vi "test_read-nmea-data2.vi"() -> ()   [LabVIEW 2019] (continued)
3,12,06,19,05,17,09,04,02,,,,,1.24,0.73,1.00,1*02\n\t\n15:12:20.33\tF9P\t$GNGSA,A,3,85,70,71,84,,,,,,,,,1.24,0.73,1.00,2*00\n\t\n15:12:20.35\tF9P\t$GNGSA,A,3,36,19,11,04,09,12,,,,,,,1.24,0.73,1.00,3*02\n\t\n15:12:20.37\tF9P\t$GNGSA,A,3,14,11,33,,,,,,,,,,1.24,0.73,1.00,4*03\n\t\n15:12:20.39\tF9P\t$GPGSV,3,1,09,02,55,319,20,04,18,043,29,05,37,247,28,06,64,049,37,1*62\n\t\n15:12:20.41\tF9P\t$GPGSV,3,2,09,09,45,074,30,12,23,276,31,17,33,154,36,19,52,157,35,1*6E\n\t\n15:12:20.43\tF9P\t$GPGSV,3,3,09,25,12,306,11,1*5C\n\t\n15:12:20.45\tF9P\t$GPGSV,3,1,09,02,55,319,,04,18,043,23,05,37,247,23,06,64,049,26,6*66\n\t\n15:12:20.47\tF9P\t$GPGSV,3,2,09,09,45,074,26,12,23,276,21,17,33,154,26,19,52,157,,6*68\n\t\n15:12:20.49\tF9P\t$GPGSV,3,3,09,25,12,306,,6*5B\n\t\n15:12:20.51\tF9P\t$GLGSV,2,1,08,69,12,031,,70,71,039,33,71,52,205,42,72,04,209,26,1*78\n\t\n15:12:20.53\tF9P\t$GLGSV,2,2,08,77,01,326,,84,20,122,08,85,70,067,40,86,37,330,,1*74\n\t\n15:12:20.55\tF9P\t$GLGSV,2,1,08,69,12,031,,70,71,039,,71,52,205,24,72,04,209,,3*7E\n\t\n15:12:20.57\tF9P\t$GLGSV,2,2,08,77,01,326,,84,20,122,13,85,70,067,23,86,37,330,,3*79\n\t\n15:12:20.59\tF9P\t$GAGSV,2,1,08,02,08,297,10,04,66,117,26,09,32,193,30,11,71,358,36,7*75\n\t\n15:12:20.61\tF9P\t$GAGSV,2,2,08,12,40,102,28,19,26,045,13,25,09,249,,36,26,308,15,7*75\n\t\n15:12:20.63\tF9P\t$GAGSV,2,1,08,02,08,297,,04,66,117,,09,32,193,,11,71,358,,2*73\n\t\n15:12:20.65\tF9P\t$GAGSV,2,2,08,12,40,102,,19,26,045,,25,09,249,,36,26,308,,2*7C\n\t\n15:12:20.67\tF9P\t$GBGSV,1,1,04,11,50,132,29,14,87,127,23,28,,,18,33,60,219,33,1*4C\n\t\n15:12:20.69\tF9P\t$GBGSV,1,1,03,11,50,132,30,14,87,127,,33,60,219,,3*43\n\t\n15:12:20.71\tF9P\t$GNGLL,3723.53875,N,12656.93680,E,061222.00,A,A*79\n\t\n15:12:20.73\tF9P\t\t\n15:12:20.75\tF9P\t\t\n15:12:20.77\tF9P\t\t\n15:12:20.79\tF9P\t\t\n15:12:20.81\tF9P\t\t\n15:12:20.83\tF9P\t\t\n15:12:20.85\tF9P\t\t\n15:12:20.87\tF9P\t\t\n15:12:20.89\tF9P\t\t\n15:12:20.91\tF9P\t\t\n15:12:20.93\tF9P\t\t\n15:12:20.95\tF9P\t\t\n15:12:20.97\tF9P\t\t\n15:12:20.99\tF9P\t\t\n15:12:21.01\tF9P\t\t\n15:12:21.03\tF9P\t\t\n15:12:21.05\tF9P\t\t\n15:12:21.07\tF9P\t\t\n15:12:21.09\tF9P\t\t\n15:12:21.11\tF9P\t\t\n15:12:21.13\tF9P\t\t\n15:12:21.15\tF9P\t\t\n15:12:21.17\tF9P\t\t\n15:12:21.19\tF9P\t\t\n15:12:21.21\tF9P\t\t\n15:12:21.23\tF9P\t\t\n15:12:21.25\tF9P\t$GNRMC,061223.00,A,3723.53919,N,12656.93709,E,1.332,46.74,250720,,,A,V*3E\n\t\n15:12:21.27\tF9P\t$GNVTG,46.74,T,,M,1.332,N,2.467,K,A*16\n\t\n15:12:21.29\tF9P\t$GNGGA,061223.00,3723.53919,N,12656.93709,E,1,12,0.86,40.3,M,18.5,M,,*70\n\t\n15:12:21.31\tF9P\t$GNGSA,A,3,12,06,19,05,17,09,04,02,,,,,1.43,0.86,1.14,1*0C\n\t\n15:12:21.33\tF9P\t$GNGSA,A,3,85,70,71,84,,,,,,,,,1.43,0.86,1.14,2*0E\n\t\n15:12:21.35\tF9P\t$GNGSA,A,3,36,19,11,04,09,12,,,,,,,1.43,0.86,1.14,3*0C\n\t\n15:12:21.37\tF9P\t$GNGSA,A,3,14,11,33,,,,,,,,,,1.43,0.86,1.14,4*0D\n\t\n15:12:21.39\tF9P\t$GPGSV,3,1,09,02,55,319,20,04,18,043,27,05,37,247,36,06,64,049,36,1*62\n\t\n15:12:21.41\tF9P\t$GPGSV,3,2,09,09,45,074,30,12,23,276,30,17,33,154,33,19,52,157,30,1*6F\n\t\n15:12:21.43\tF9P\t$GPGSV,3,3,09,25,12,306,,1*5C\n\t\n15:12:21.45\tF9P\t$GPGSV,3,1,09,02,55,319,,04,18,043,22,05,37,247,24,06,64,049,27,6*61\n\t\n15:12:21.47\tF9P\t$GPGSV,3,2,09,09,45,074,25,12,23,276,20,17,33,154,25,19,52,157,,6*69\n\t\n15:12:21.49\tF9P\t$GPGSV,3,3,09,25,12,306,,6*5B\n\t\n15:12:21.51\tF9P\t$GLGSV,2,1,08,69,12,031,,70,71,039,30,71,52,205,39,72,04,209,25,1*74\n\t\n15:12:21.53\tF9P\t$GLGSV,2,2,08,77,01,326,,84,20,122,12,85,70,067,33,86,37,330,,1*7B\n\t\n15:12:21.55\tF9P\t$GLGSV,2,1,08,69,12,031,,70,71,039,,71,52,205,25,72,04,209,,3*7F\n\t\n15:12:21.57\tF9P\t$GLGSV,2,2,08,77,01,326,,84,20,122,12,85,70,067,21,86,37,330,,3*7A\n\t\n15:12:21.59\tF9P\t$GAGSV,2,1,08,02,08,297,08,04,66,117,34,09,32,193,30,11,71,358,37,7*7E\n\t\n15:12:21.61\tF9P\t$GAGSV,2,2,08,12,40,102,29,19,26,045,12,25,09,249,,36,26,308,14,7*74\n\t\n15:12:21.63\tF9P\t$GAGSV,2,1,08,02,08,297,,04,66,117,,09,32,193,,11,71,358,32,2*72\n\t\n15:12:21.65\tF9P\t$GAGSV,2,2,08,12,40,102,,19,26,045,,25,09,249,,36,26,308,,2*7C\n\t\n15:12:21.67\tF9P\t$GBGSV,1,1,04,11,50,132,28,14,87,127,24,28,,,17,33,60,219,33,1*45\n\t\n15:12:21.69\tF9P\t$GBGSV,1,1,03,11,50,132,,14,87,127,,33,60,219,,3*40\n\t\n15:12:21.71\tF9P\t$GNGLL,3723.53919,N,12656.93709,E,061223.00,A,A*73\n\t\n15:12:21.73\tF9P\t\t\n15:12:21.75\tF9P\t\t\n15:12:21.77\tF9P\t\t\n15:12:21.79\tF9P\t\t\n15:12:21.81\tF9P\t\t\n15:12:21.83\tF9P\t\t\n15:12:21.85\tF9P\t\t\n15:12:21.87\tF9P\t\t\n15:12:21.89\tF9P\t\t\n15:12:21.91\tF9P\t\t\n15:12:21.93\tF9P\t\t\n15:12:21.95\tF9P\t\t\n15:12:21.97\tF9P\t\t\n15:12:21.99\tF9P\t\t\n15:12:22.01\tF9P\t\t\n15:12:22.03\tF9P\t\t\n15:12:22.05\tF9P\t\t\n15:12:22.07\tF9P\t\t\n15:12:22.09\tF9P\t\t\n15:12:22.11\tF9P\t\t\n15:12:22.13\tF9P\t\t\n15:12:22.15\tF9P\t\t\n15:12:22.17\tF9P\t\t\n15:12:22.19\tF9P\t\t\n15:12:22.21\tF9P\t\t\n15:12:22.23\tF9P\t$GNRMC,061224.00,A,3723.53944,N,12656.93745,E,1.337,51.42,250720\t\n15:12:22.25\tF9P\t,,,A,V*3F\n\t\n15:12:22.27\tF9P\t$GNVTG,51.42,T,,M,1.337,N,2.476,K,A*10\n\t\n15:12:22.29\tF9P\t$GNGGA,061224.00,3723.53944,N,12656.93745,E,1,12,0.73,40.9,M,18.5,M,,*77\n\t\n15:12:22.31\tF9P\t$GNGSA,A,3,12,06,19,05,17,09,04,02,,,,,1.26,0.73,1.03,1*03\n\t\n15:12:22.33\tF9P\t$GNGSA,A,3,85,70,71,84,,,,,,,,,1.26,0.73,1.03,2*01\n\t\n15:12:22.35\tF9P\t$GNGSA,A,3,36,19,11,04,09,12,,,,,,,1.26,0.73,1.03,3*03\n\t\n15:12:22.37\tF9P\t$GNGSA,A,3,14,11,33,,,,,,,,,,1.26,0.73,1.03,4*02\n\t\n15:12:22.39\tF9P\t$GPGSV,3,1,09,02,55,319,20,04,18,043,31,05,37,247,31,06,64,049,28,1*6D\n\t\n15:12:22.41\tF9P\t$GPGSV,3,2,09,09,45,074,28,12,23,276,30,17,33,154,30,19,52,157,36,1*63\n\t\n15:12:22.43\tF9P\t$GPGSV,3,3,09,25,12,306,,1*5C\n\t\n15:12:22.45\tF9P\t$GPGSV,3,1,09,02,55,319,,04,18,043,20,05,37,247,24,06,64,049,26,6*62\n\t\n15:12:22.47\tF9P\t$GPGSV,3,2,09,09,45,074,25,12,23,276,19,17,33,154,26,19,52,157,,6*60\n\t\n15:12:22.49\tF9P\t$GPGSV,3,3,09,25,12,306,,6*5B\n\t\n15:12:22.51\tF9P\t$GLGSV,2,1,08,69,12,031,,70,71,039,33,71,52,205,30,72,04,209,23,1*78\n\t\n15:12:22.53\tF9P\t$GLGSV,2,2,08,77,01,326,,84,20,122,10,85,70,067,35,86,37,330,,1*7F\n\t\n15:12:22.55\tF9P\t$GLGSV,2,1,08,69,12,031,,70,71,039,,71,52,205,24,72,04,209,,3*7E\n\t\n15:12:22.57\tF9P\t$GLGSV,2,2,08,77,01,326,,84,20,122,11,85,70,067,21,86,37,330,,3*79\n\t\n15:12:22.59\tF9P\t$GAGSV,2,1,08,02,08,297,07,04,66,117,31,09,32,193,31,11,71,358,37,7*75\n\t\n15:12:22.61\tF9P\t$GAGSV,2,2,08,12,40,102,29,19,26,045,11,25,09,249,,36,26,308,14,7*77\n\t\n15:12:22.63\tF9P\t$GAGSV,2,1,08,02,08,297,,04,66,117,29,09,32,193,,11,71,358,,2*78\n\t\n15:12:22.65\tF9P\t$GAGSV,2,2,08,12,40,102,,19,26,045,,25,09,249,,36,26,308,,2*7C\n\t\n15:12:22.67\tF9P\t$GBGSV,1,1,04,11,50,132,29,14,87,127,30,28,,,18,33,60,219,29,1*45\n\t\n15:12:22.69\tF9P\t$GBGSV,1,1,03,11,50,132,29,14,87,127,,33,60,219,,3*4B\n\t\n15:12:22.71\tF9P\t$GNGLL,3723.53944,N,12656.93745,E,061224.00,A,A*74\n\t\n15:12:22.73\tF9P\t\t\n15:12:22.75\tF9P\t\t\n15:12:22.77\tF9P\t\t\n15:12:22.79\tF9P\t\t\n15:12:22.81\tF9P\t\t\n15:12:22.83\tF9P\t\t\n15:12:22.85\tF9P\t\t\n15:12:22.87\tF9P\t\t\n15:12:22.89\tF9P\t\t\n15:12:22.91\tF9P\t\t\n15:12:22.93\tF9P\t\t\n15:12:22.95\tF9P\t\t\n15:12:22.97\tF9P\t\t\n15:12:22.99\tF9P\t\t\n15:12:23.01\tF9P\t\t\n15:12:23.03\tF9P\t\t\n15:12:23.05\tF9P\t\t\n15:12:23.07\tF9P\t\t\n15:12:23.09\tF9P\t\t\n15:12:23.11\tF9P\t\t\n15:12:23.13\tF9P\t\t\n15:12:23.15\tF9P\t\t\n15:12:23.17\tF9P\t\t\n15:12:23.19\tF9P\t\t\n15:12:23.21\tF9P\t\t\n15:12:23.23\tF9P\t$GNRMC,061225.00,A,3723.53964,N,12656.93801,E,1.830,59.59,250720,,,A,V*3D\n\t\n15:12:23.25\tF9P\t$GNVTG,59.59,T,,M,1.830,N,3.389,K,A*18\n\t\n15:12:23.27\tF9P\t$GNGGA,061225.00,3723.53964,N,12656.93801,E,1,12,0.74,41.4,M,18.5,M,,*70\n\t\n15:12:23.29\tF9P\t$GNGSA,A,3,12,06,19,05,17,09,04,02,,,,,1.27,0.74,1.04,1*02\n\t\n15:12:23.31\tF9P\t$GNGSA,A,3,85,70,71,84,,,,,,,,,1.27,0.74,1.04,2*00\n\t\n15:12:23.33\tF9P\t$GNGSA,A,3,36,19,11,04,09,12,,,,,,,1.27,0.74,1.04,3*02\n\t\n15:12:23.35\tF9P\t$GNGSA,A,3,14,11,33,,,,,,,,,,1.27,0.74,1.04,4*03\n\t\n15:12:23.37\tF9P\t$GPGSV,3,1,09,02,55,319,21,04,18,043,24,05,37,247,27,06,64,049,29,1*6E\n\t\n15:12:23.39\tF9P\t$GPGSV,3,2,09,09,45,074,34,12,23,276,29,17,33,154,32,19,52,157,32,1*60\n\t\n15:12:23.41\tF9P\t$GPGSV,3,3,09,25,12,306,,1*5C\n\t\n15:12:23.43\tF9P\t$GPGSV,3,1,09,02,55,319,,04,18,043,21,05,37,247,24,06,64,049,26,6*63\n\t\n15:12:23.45\tF9P\t$GPGSV,3,2,09,09,45,074,26,12,23,276,19,17,33,154,25,19,52,157,,6*60\n\t\n15:12:23.47\tF9P\t$GPGSV,3,3,09,25,12,306,,6*5B\n\t\n15:12:23.49\tF9P\t$GLGSV,2,1,08,69,12,031,,70,71,039,29,71,52,205,40,72,04,209,24,1*73\n\t\n15:12:23.51\tF9P\t$GLGSV,2,2,08,77,01,326,,84,20,122,08,85,70,067,34,86,37,330,,1*77\n\t\n15:12:23.53\tF9P\t$GLGSV,2,1,08,69,12,031,,70,71,039,,71,52,205,23,72,04,209,,3*79\n\t\n15:12:23.55\tF9P\t$GLGSV,2,2,08,77,01,326,,84,20,122,11,85,70,067,23,86,37,330,,3*7B\n\t\n15:12:23.57\tF9P\t$GAGSV,2,1,08,02,08,297,12,04,66,117,31,09,32,193,35,11,71,358,32,7*70\n\t\n15:12:23.59\tF9P\t$GAGSV,2,2,08,12,40,102,29,19,26,045,11,25,09,249,,36,26,308,15,7*76\n\t\n15:12:23.61\tF9P\t$GAGSV,2,1,08,02,08,297,,04,66,117,,09,32,193,,11,71,358,33,2*73\n\t\n15:12:23.63\tF9P\t$GAGSV,2,2,08,12,40,102,,19,26,045,,25,09,249,,36,26,308,,2*7C\n\t\n15:12:23.65\tF9P\t$GBGSV,1,1,04,11,50,132,29,14,87,127,30,28,,,18,33,60,219,33,1*4E\n\t\n15:12:23.67\tF9P\t$GBGSV,1,1,03,11,50,132,,14,87,127,,33,60,219,,3*40\n\t\n15:12:23.69\tF9P\t$GNGLL,3723.53964,N,12656.93801,E,061225.00,A,A*78\n\t\n15:12:23.71\tF9P\t\t\n15:12:23.73\tF9P\t\t\n15:12:23.75\tF9P\t\t\n15:12:23.77\tF9P\t\t\n15:12:23.79\tF9P\t\t\n15:12:23.81\tF9P\t\t\n15:12:23.83\tF9P\t\t\n15:12:23.85\tF9P\t\t\n15:12:23.87\tF9P\t\t\n15:12:23.89\tF9P\t\t\n15:12:23.91\tF9P\t\t\n15:12:23.93\tF9P\t\t\n15:12:23.95\tF9P\t\t\n15:12:23.97\tF9P\t\t\n15:12:23.99\tF9P\t\t\n15:12:24.01\tF9P\t\t\n15:12:24.03\tF9P\t\t\n15:12:24.05\tF9P\t\t\n15:12:24.07\tF9P\t\t\n15:12:24.09\tF9P\t\t\n15:12:24.11\tF9P\t\t\n15:12:24.13\tF9P\t\t\n15:12:24.15\tF9P\t\t\n15:12:24.17\tF9P\t\t\n15:12:24.19\tF9P\t\t\n15:12:24.21\tF9P\t\t\n15:12:24.23\tF9P\t$GNRMC,061226.00,A,3723.53985,N,12656.93886,E,2.379,68.89,250720,,,A,V*34\n\t\n15:12:24.25\tF9P\t$GNVTG,68.89,T,,M,2.379,N,4.406,K,A*15\n\t\n15:12:24.27\tF9P\t$GNGGA,061226.00,3723.53985,N,12656.93886,E,1,12,0.73,41.5,M,18.5,M,,*75\n\t\n15:12:24.29\tF9P\t$GNGSA,A,3,12,06,19,05,17,09,04,02,,,,,1.24,0.73,1.00,1*02\n\t\n15:12:24.31\tF9P\t$GNGSA,A,3,85,70,71,84,,,,,,,,,1.24,0.73,1.00,2*00\n\t\n15:12:24.33\tF9P\t$GNGSA,A,3,36,19,11,04,09,12,,,,,,,1.24,0.73,1.00,3*02\n\t\n15:12:24.35\tF9P\t$GNGSA,A,3,14,11,33,,,,,,,,,,1.24,0.73,1.00,4*03\n\t\n15:12:24.37\tF9P\t$GPGSV,3,1,09,02,55,319,20,04,18,043,26,05,37,247,33,06,64,049,29,1*68\n\t\n15:12:24.39\tF9P\t$GPGSV,3,2,09,09,45,074,29,12,23,276,28,17,33,154,35,19,52,157,32,1*6A\n\t\n15:12:24.41\tF9P\t$GPGSV,3,3,09,25,12,306,,1*5C\n\t\n15:12:24.43\tF9P\t$GPGSV,3,1,09,02,55,319,,04,18,043,22,05,37,247,24,06,64,049,27,6*61\n\t\n15:12:24.45\tF9P\t$GPGSV,3,2,09,09,45,074,31,12,23,276,19,17,33,154,27,19,52,157,,6*64\n\t\n15:12:24.47\tF9P\t$GPGSV,3,3,09,25,12,306,,6*5B\n\t\n15:12:24.49\tF9P\t$GLGSV,2,1,08,69,12,031,,70,71,039,29,71,52,205,43,72,04,209,25,1*71\n\t\n15:12:24.51\tF9P\t$GLGSV,2,2,08,77,01,326,,84,20,122,12,85,70,067,35,86,37,330,,1*7D\n\t\n15:12:24.53\tF9P\t$GLGSV,2,1,08,69,12,031,,70,71,039,,71,52,205,30,72,04,209,,3*7B\n\t\n15:12:24.55\tF9P\t$GLGSV,2,2,08,77,01,326,,84,20,122,11,85,70,067,22,86,37,330,,3*7A\n\t\n15:12:24.57\tF9P\t$GAGSV,2,1,08,02,08,297,10,04,66,117,30,09,32,193,38,11,71,358,32,7*7E\n\t\n15:12:24.59\tF9P\t$GAGSV,2,2,08,12,40,102,29,19,26,045,13,25,09,249,,36,26,308,15,7*74\n\t\n15:12:24.61\tF9P\t$GAGSV,2,1,08,02,08,297,,04,66,117,,09,32,193,,11,71,358,,2*73\n\t\n15:12:24.63\tF9P\t$GAGSV,2,2,08,12,40,102,,19,26,045,,25,09,249,,36,26,308,,2*7C\n\t\n15:12:24.65\tF9P\t$GBGSV,1,1,04,11,50,132,30,14,87,127,30,28,,,18,33,60,219,28,1*4C\n\t\n15:12:24.67\tF9P\t$GBGSV,1,1,03,11,50,132,,14,87,127,,33,60,219,,3*40\n\t\n15:12:24.69\tF9P\t$GNGLL,3723.53985,N,12656.93886,E,061226.00,A,A*7B\n\t\n15:12:24.71\tF9P\t\t\n15:12:24.73\tF9P\t\t\n15:12:24.75\tF9P\t\t\n15:12:24.77\tF9P\t\t\n15:12:24.79\tF9P\t\t\n15:12:24.81\tF9P\t\t\n15:12:24.83\tF9P\t\t\n15:12:24.85\tF9P\t\t\n15:12:24.87\tF9P\t\t\n15:12:24.89\tF9P\t\t\n15:12:24.91\tF9P\t\t\n15:12:24.93\tF9P\t\t\n15:12:24.95\tF9P\t\t\n15:12:24.97\tF9P\t\t\n15:12:24.99\tF9P\t\t\n15:12:25.01\tF9P\t\t\n15:12:25.03\tF9P\t\t\n15:12:25.05\tF9P\t\t\n15:12:25.07\tF9P\t\t\n15:12:25.09\tF9P\t\t\n15:12:25.11\tF9P\t\t\n15:12:25.13\tF9P\t\t\n15:12:25.15\tF9P\t\t\n15:12:25.17\tF9P\t\t\n15:12:25.19\tF9P\t\t\n15:12:25.21\tF9P\t\t\n15:12:25.23\tF9P\t$GNRMC,061227.00,A,3723.53985,N,12656.93969,E,2.036,75.18,250720,,,A,V*39\n\t\n15:12:25.25\tF9P\t$GNVTG,75.18,T,,M,2.036,N,3.770,K,A*1C\n\t\n15:12:25.27\tF9P\t$GNGGA,061227.00,3723.53985,N,12656.93969,E,1,12,0.93,41.9,M,18.5,M,,*76\n\t\n15:12:25.29\tF9P\t$GNGSA,A,3,12,06,19,05,17,09,04,02,,,,,1.55,0.93,1.24,1*0C\n\t\n15:12:25.31\tF9P\t$GNGSA,A,3,85,70,71,84,,,,,,,,,1.55,0.93,1.24,2*0E\n\t\n15:12:25.33\tF9P\t$GNGSA,A,3,36,19,11,04,09,12,,,,,,,1.55,0.93,1.24,3*0C\n\t\n15:12:25.35\tF9P\t$GNGSA,A,3,14,11,33,,,,,,,,,,1.55,0.93,1.24,4*0D\n\t\n15:12:25.37\tF9P\t$GPGSV,3,1,09,02,55,319,20,04,18,043,26,05,37,247,36,06,64,049,33,1*66\n\t\n15:12:25.39\tF9P\t$GPGSV,3,2,09,09,45,074,28,12,23,276,28,17,33,154,34,19,52,157,32,1*6A\n\t\n15:12:25.41\tF9P\t$GPGSV,3,3,09,25,12,306,,1*5C\n\t\n15:12:25.43\tF9P\t$GPGSV,3,1,09,02,55,319,,04,18,043,21,05,37,247,25,06,64,049,26,6*62\n\t\n15:12:25.45\tF9P\t$GPGSV,3,2,09,09,45,074,23,12,23,276,21,17,33,154,27,19,52,157,,6*6C\n\t\n15:12:25.47\tF9P\t$GPGSV,3,3,09,25,12,306,,6*5B\n\t\n15:12:25.49\tF9P\t$GLGSV,2,1,08,69,12,031,,70,71,039,29,71,52,205,42,72,04,209,26,1*73\n\t\n15:12:25.51\tF9P\t$GLGSV,2,2,08,77,01,326,,84,20,122,10,85,70,067,32,86,37,330,,1*78\n\t\n15:12:25.53\tF9P\t$GLGSV,2,1,08,69,12,031,,70,71,039,,71,52,205,30,72,04,209,,3*7B\n\t\n15:12:25.55\tF9P\t$GLGSV,2,2,08,77,01,326,,84,20,122,09,85,70,067,23,86,37,330,,3*72\n\t\n15:12:25.57\tF9P\t$GAGSV,2,1,08,02,08,297,10,04,66,116,29,09,32,193,38,11,71,358,27,7*73\n\t\n15:12:25.59\tF9P\t$GAGSV,2,2,08,12,40,102,30,19,26,045,15,25,09,249,,36,26,308,14,7*7B\n\t\n15:12:25.61\tF9P\t$GAGSV,2,1,08,02,08,297,,04,66,116,,09,32,193,,11,71,358,,2*72\n\t\n15:12:25.63\tF9P\t$GAGSV,2,2,08,12,40,102,,19,26,045,,25,09,249,,36,26,308,,2*7C\n\t\n15:12:25.65\tF9P\t$GBGSV,1,1,04,11,50,132,28,14,87,127,30,28,,,18,33,60,219,28,1*45\n\t\n15:12:25.67\tF9P\t$GBGSV,1,1,03,11,50,132,,14,87,127,,33,60,219,,3*40\n\t\n15:12:25.69\tF9P\t$GNGLL,3723.53985,N,12656.93969,E,061227.00,A,A*7A\n\t\n15:12:25.71\tF9P\t\t\n15:12:25.73\tF9P\t\t\n15:12:25.75\tF9P\t\t\n15:12:25.77\tF9P\t\t\n15:12:25.79\tF9P\t\t\n15:12:25.81\tF9P\t\t\n15:12:25.83\tF9P\t\t\n15:12:25.85\tF9P\t\t\n15:12:25.87\tF9P\t\t\n15:12:25.89\tF9P\t\t\n15:12:25.91\tF9P\t\t\n15:12:25.93\tF9P\t\t\n15:12:25.95\tF9P\t\t\n15:12:25.97\tF9P\t\t\n15:12:25.99\tF9P\t\t\n15:12:26.01\tF9P\t\t\n15:12:26.03\tF9P\t\t\n15:12:26.05\tF9P\t\t\n15:12:26.07\tF9P\t\t\n15:12:26.09\tF9P\t\t\n15:12:26.11\tF9P\t\t\n15:12:26.13\tF9P\t\t\n15:12:26.15\tF9P\t\t\n15:12:26.17\tF9P\t\t\n15:12:26.19\tF9P\t\t\n15:12:26.21\tF9P\t\t\n15:12:26.23\tF9P\t$GNRMC,061228.00,A,3723.54009,N,12656.94073,E,2.854,71.20,250720,,,A,V*3A\n\t\n15:12:26.25\tF9P\t$GNVTG,71.20,T,,M,2.854,N,5.286,K,A*15\n\t\n15:12:26.27\tF9P\t$GNGGA,061228.00,3723.54009,N,12656.94073,E,1,12,0.75,41.7,M,18.5,M,,*70\n\t\n15:12:26.29\tF9P\t$GNGSA,A,3,12,06,19,05,17,09,04,02,,,,,1.29,0.75,1.04,1*0D\n\t\n15:12:26.31\tF9P\t$GNGSA,A,3,85,70,71,84,,,,,,,,,1.29,0.75,1.04,2*0F\n\t\n15:12:26.33\tF9P\t$GNGSA,A,3,36,19,11,04,09,12,,,,,,,1.29,0.75,1.04,3*0D\n\t\n15:12:26.35\tF9P\t$GNGSA,A,3,14,11,33,,,,,,,,,,1.29,0.75,1.04,4*0C\n\t\n15:12:26.37\tF9P\t$GPGSV,3,1,09,02,55,319,20,04,18,043,25,05,37,247,44,06,64,049,30,1*63\n\t\n15:12:26.39\tF9P\t$GPGSV,3,2,09,09,45,074,27,12,23,276,27,17,33,154,34,19,52,157,26,1*6F\n\t\n15:12:26.41\tF9P\t$GPGSV,3,3,09,25,12,306,,1*5C\n\t\n15:12:26.43\tF9P\t$GPGSV,3,1,09,02,55,319,,04,18,043,21,05,37,247,25,06,64,049,26,6*62\n\t\n15:12:26.45\tF9P\t$GPGSV,3,2,09,09,45,074,25,12,23,276,21,17,33,154,27,19,52,157,,6*6A\n\t\n15:12:26.47\tF9P\t$GPGSV,3,3,09,25,12,306,,6*5B\n\t\n15:12:26.49\tF9P\t$GLGSV,2,1,08,69,12,031,,70,71,039,27,71,52,205,45,72,04,209,24,1*78\n\t\n15:12:26.51\tF9P\t$GLGSV,2,2,08,77,01,326,,84,20,122,08,85,70,067,29,86,37,330,,1*7B\n\t\n15:12:26.53\tF9P\t$GLGSV,2,1,08,69,12,031,,70,71,039,,71,52,205,24,72,04,209,,3*7E\n\t\n15:12:26.55\tF9P\t$GLGSV,2,2,08,77,01,326,,84,20,122,13,85,70,067,24,86,37,330,,3*7E\n\t\n15:12:26.57\tF9P\t$GAGSV,2,1,08,02,08,297,07,04,66,116,29,09,32,193,40,11,71,358,26,7*7B\n\t\n15:12:26.59\tF9P\t$GAGSV,2,2,08,12,40,102,30,19,26,045,15,25,09,249,,36,26,308,15,7*7A\n\t\n15:12:26.61\tF9P\t$GAGSV,2,1,08,02,08,297,,04,66,116,,09,32,193,,11,71,358,,2*72\n\t\n15:12:26.63\tF9P\t$GAGSV,2,2,08,12,40,102,,19,26,045,,25,09,249,,36,26,308,,2*7C\n\t\n15:12:26.65\tF9P\t$GBGSV,1,1,04,11,50,132,28,14,87,127,28,28,,,18,33,60,219,38,1*4D\n\t\n15:12:26.67\tF9P\t$GBGSV,1,1,03,11,50,132,,14,87,127,,33,60,219,,3*40\n\t\n15:12:26.69\tF9P\t$GNGLL,3723.54009,N,12656.94073,E,061228.00,A,A*7A\n\t\n15:12:26.71\tF9P\t\t\n15:12:26.73\tF9P\t\t\n15:12:26.75\tF9P\t\t\n15:12:26.77\tF9P\t\t\n15:12:26.79\tF9P\t\t\n15:12:26.81\tF9P\t\t\n15:12:26.83\tF9P\t\t\n15:12:26.85\tF9P\t\t\n15:12:26.87\tF9P\t\t\n15:12:26.89\tF9P\t\t\n15:12:26.91\tF9P\t\t\n15:12:26.93\tF9P\t\t\n15:12:26.95\tF9P\t\t\n15:12:26.97\tF9P\t\t\n15:12:26.99\tF9P\t\t\n15:12:27.01\tF9P\t\t\n15:12:27.03\tF9P\t\t\n15:12:27.05\tF9P\t\t\n15:12:27.07\tF9P\t\t\n15:12:27.09\tF9P\t\t\n15:12:27.11\tF9P\t\t\n15:12:27.13\tF9P\t\t\n15:12:27.15\tF9P\t\t\n15:12:27.17\tF9P\t\t\n15:12:27.19\tF9P\t\t\n15:12:27.21\tF9P\t\t\n15:12:27.23\tF9P\t$GNRMC,061229.00,A,3723.54017,N,12656.94177,E,2.235,67.59,250720,,,A,V*35\n\t\n15:12:27.25\tF9P\t$GNVTG,67.59,T,,M,2.235,N,4.139,K,A*17\n\t\n15:12:27.27\tF9P\t$GNGGA,061229.00,3723.54017,N,12656.94177,E,1,12,0.75,42.1,M,18.5,M,,*7E\n\t\n15:12:27.29\tF9P\t$GNGSA,A,3,12,06,19,05,17,09,04,02,,,,,1.29,0.75,1.04,1*0D\n\t\n15:12:27.31\tF9P\t$GNGSA,A,3,85,70,71,84,,,,,,,,,1.29,0.75,1.04,2*0F\n\t\n15:12:27.33\tF9P\t$GNGSA,A,3,36,19,11,04,09,12,,,,,,,1.29,0.75,1.04,3*0D\n\t\n15:12:27.35\tF9P\t$GNGSA,A,3,14,11,33,,,,,,,,,,1.29,0.75,1.04,4*0C\n\t\n15:12:27.37\tF9P\t$GPGSV,3,1,09,02,55,319,19,04,18,043,25,05,37,247,39,06,64,049,34,1*67\n\t\n15:12:27.39\tF9P\t$GPGSV,3,2,09,09,45,074,35,12,23,276,27,17,33,154,28,19,52,157,32,1*64\n\t\n15:12:27.41\tF9P\t$GPGSV,3,3,09,25,12,306,,1*5C\n\t\n15:12:27.43\tF9P\t$GPGSV,3,1,09,02,55,319,,04,18,043,21,05,37,247,26,06,64,049,27,6*60\n\t\n15:12:27.45\tF9P\t$GPGSV,3,2,09,09,45,074,27,12,23,276,19,17,33,154,26,19,52,157,,6*62\n\t\n15:12:27.47\tF9P\t$GPGSV,3,3,09,25,12,306,,6*5B\n\t\n15:12:27.49\tF9P\t$GLGSV,2,1,08,69,12,031,,70,71,039,28,71,52,205,45,72,04,209,23,1*70\n\t\n15:12:27.51\tF9P\t$GLGSV,2,2,08,77,01,326,,84,20,122,11,85,70,067,29,86,37,330,,1*73\n\t\n15:12:27.53\tF9P\t$GLGSV,2,1,08,69,12,031,,70,71,039,,71,52,205,32,72,04,209,,3*79\n\t\n15:12:27.55\tF9P\t$GLGSV,2,2,08,77,01,326,,84,20,122,12,85,70,067,24,86,37,330,,3*7F\n\t\n15:12:27.57\tF9P\t$GAGSV,2,1,08,02,08,297,09,04,66,116,29,09,32,193,38,11,71,358,28,7*74\n\t\n15:12:27.59\tF9P\t$GAGSV,2,2,08,12,40,102,32,19,26,045,15,25,09,249,,36,26,308,14,7*79\n\t\n15:12:27.61\tF9P\t$GAGSV,2,1,08,02,08,297,,04,66,116,,09,32,193,,11,71,358,,2*72\n\t\n15:12:27.63\tF9P\t$GAGSV,2,2,08,12,40,102,,19,26,045,,25,09,249,,36,26,308,,2*7C\n\t\n15:12:27.65\tF9P\t$GBGSV,1,1,04,11,50,132,28,14,87,127,27,28,,,17,33,60,219,35,1*40\n\t\n15:12:27.67\tF9P\t$GBGSV,1,1,03,11,50,132,,14,87,127,,33,60,219,,3*40\n\t\n15:12:27.69\tF9P\t$GNGLL,3723.54017,N,12656.94177,E,061229.00,A,A*71\n\t\n15:12:27.71\tF9P\t\t\n15:12:27.73\tF9P\t\t\n15:12:27.75\tF9P\t\t\n15:12:27.77\tF9P\t\t\n15:12:27.79\tF9P\t\t\n15:12:27.81\tF9P\t\t\n15:12:27.83\tF9P\t\t\n15:12:27.85\tF9P\t\t\n15:12:27.87\tF9P\t\t\n15:12:27.89\tF9P\t\t\n15:12:27.91\tF9P\t\t\n15:12:27.93\tF9P\t\t\n15:12:27.95\tF9P\t\t\n15:12:27.97\tF9P\t\t\n15:12:27.99\tF9P\t\t
